vi "get hot pixel correction status.vi"(8 "error in (no error)":errorcluster, 11 "Thorcam in":refnum<class "Thorcam.lvclass">) -> (0 "error out":errorcluster, 3 "Thorcam out":refnum<class "Thorcam.lvclass">)   [LabVIEW 2012, in "Thorcam.lvclass"]
uses:
  Thorcam.lvclass
panel:
  out "Value":i32
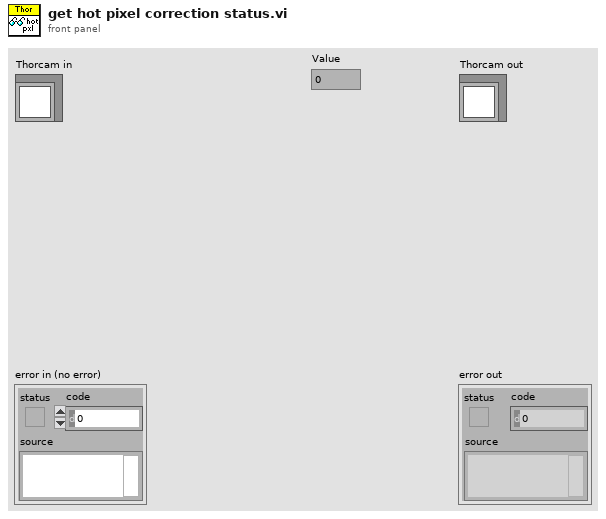
[diagram p1: front panel]
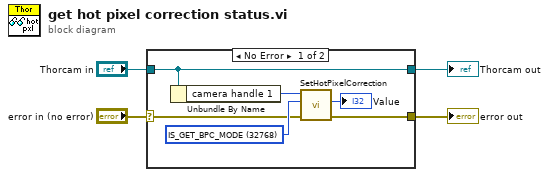
[diagram p0: block diagram]
diagram:
  n1 = case shown="No Error" "error in (no error)" {
    selector: "error in (no error)" -> [w7 w12]
    tunnel: [w6 w12] -> w3
    tunnel: [w10 w11] -> w1
    tunnel: "Thorcam in" -> [w10 w11]
    frame No Error {
      w8 = 32768 items=["IS_BPC_DISABLE"=0, "IS_BPC_ENABLE_SOFTWARE"=2, "IS_GET_BPC_MODE"=32768] ("Mode")
      n2 = Unbundle By Name(w10) -> ("camera handle 1"=w9:u32)
      n3 = call <instrlib>:"SetHotPixelCorrection.vi"("error in"=w7, "Mode"=w8, "Camera Handle In"=w9) -> ("error out"=w6:errorcluster, "Value"=→"Value":i32)  [unwired: 6 in, 1 out]
    }
    frame Error {
    }
  }
  "error out" <- w3
  "Thorcam out" <- w1
